vi "Data_folder_Path.vi"(1 "seconds":dbl, 2 "Data Type":string="Colour Calib") -> (0 "Data Folder":path)   [LabVIEW 2010]
uses:
  Globals/Constants_global.vi
  Globals/Preference_global.vi
panel:
  out "Hierarchy":string[](array[string])
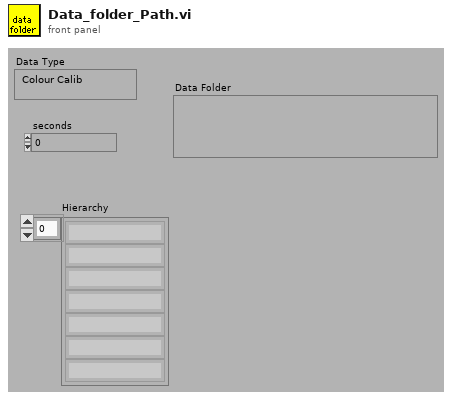
[diagram p1: front panel]
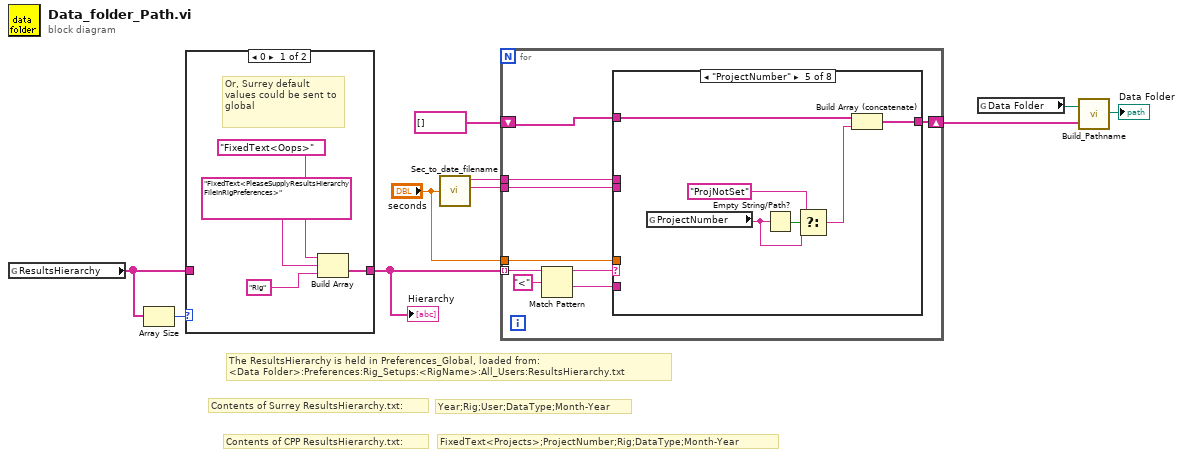
[diagram p0: block diagram]
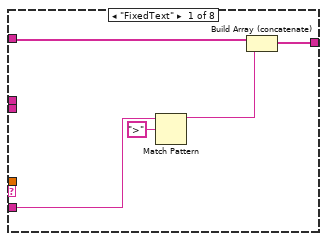
[diagram p3: hidden frame]
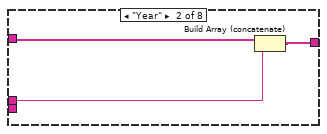
[diagram p4: hidden frame]
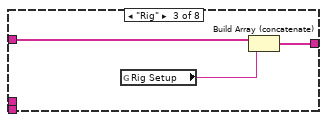
[diagram p5: hidden frame]
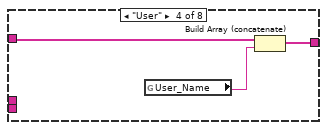
[diagram p6: hidden frame]
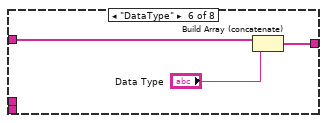
[diagram p7: hidden frame]
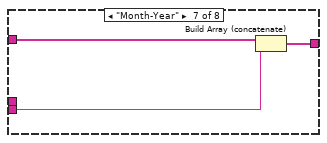
[diagram p8: hidden frame]
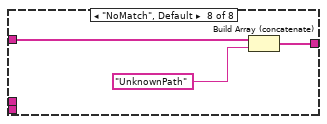
[diagram p9: hidden frame]
diagram:
  # "The ResultsHierarchy is held in Preferences_Global, loaded from:\n<Data Folder>:Preferences:Rig_Setups:<RigName>:All_Users:ResultsHierarchy.txt"
  # "Contents of CPP ResultsHierarchy.txt:"
  # "Contents of Surrey ResultsHierarchy.txt:"
  # "Year;Rig;User;DataType;Month-Year"
  # "FixedText<Projects>;ProjectNumber;Rig;DataType;Month-Year"
  n1 = global read "Preference_global.vi" "ResultsHierarchy"() -> (w1:string[])
  n2 = Array Size(array=w1) -> (size(s)=w3:i32)
  n3 = case shown="0" w3 {
    tunnel: [w14 w15] -> w2
    tunnel: w1 -> [_ w15]
    frame 0 {
      # "Or, Surrey default values could be sent to global"
      n4 = Build Array("FixedText<Oops>" ("element"), "FixedText<PleaseSupplyResultsHierarchyFileInRigPreferences>" ("element"), "Rig" ("element")) -> (w14:string[])
    }
    frame 1, Default {
    }
  }
  "Hierarchy" <- w2
  n5 = call "Sec_to_date_filename.vi"("seconds"="seconds") -> ("Year"=w6:string, "Month"=w7:string)  [unwired: 2 out]
  n6 = for {
    shift-right: [w24] -> w8
    shift-left: string[] [] -> [w23]
    tunnel: w2 -> [w19] mode=indexing
    tunnel: w7 -> [w22]
    tunnel: w6 -> [w21]
    tunnel: "seconds" -> [w20]
    n7 = Match Pattern(string=w19, regular expression="<") -> (before substring=w18:string, after substring=w16:string)  [unwired: 1 in, 2 out]
    n8 = case shown="\"ProjectNumber\"" w18 {
      tunnel: [w29 w32 w34 w38 w44 w47 w50 w53] -> w24
      tunnel: w23 -> [w28 w31 w33 w36 w43 w46 w49 w52]
      tunnel: w22 -> [_ _ _ _ _ _ w48 _]
      tunnel: w21 -> [_ w30 _ _ _ _ _ _]
      tunnel: w20 -> [_ _ _ _ _ _ _ _]
      tunnel: w16 -> [w27 _ _ _ _ _ _ _]
      frame "FixedText" {
        n9 = Match Pattern(string=w27, regular expression=">") -> (before substring=w25:string)  [unwired: 1 in, 3 out]
        n10 = Build Array (concatenate)(w28, w25) -> (w29:string[])
      }
      frame "Year" {
        n11 = Build Array (concatenate)(w31, w30) -> (w32:string[])
      }
      frame "Rig" {
        n12 = global read "Preference_global.vi" "Rig Setup"() -> (w35:string)
        n13 = Build Array (concatenate)(w33, w35) -> (w34:string[])
      }
      frame "User" {
        n14 = global read "Preference_global.vi" "User_Name"() -> (w37:string)
        n15 = Build Array (concatenate)(w36, w37) -> (w38:string[])
      }
      frame "ProjectNumber" {
        n16 = global read "Preference_global.vi" "ProjectNumber"() -> (w40:string)
        n17 = Empty String/Path?(string/path=w40) -> (empty?=w42:bool)
        n18 = Select(t="ProjNotSet", s=w42, f=w40) -> (s? t:f=w41:string)
        n19 = Build Array (concatenate)(w43, w41) -> (w44:string[])
      }
      frame "DataType" {
        n20 = Build Array (concatenate)(w46, "Data Type") -> (w47:string[])
      }
      frame "Month-Year" {
        n21 = Build Array (concatenate)(w49, w48) -> (w50:string[])
      }
      frame "NoMatch", Default {
        n22 = Build Array (concatenate)(w52, "UnknownPath" ("element")) -> (w53:string[])
      }
    }
  }
  n23 = global read "Constants_global.vi" "Data Folder"() -> (w10:path)
  n24 = call "Build_Pathname.vi"("Output Array"=w8, "Pathname"=w10) -> ("Appended path"=→"Data Folder":path)
